vi "Day 23.vi"() -> ()   [LabVIEW 2021]
uses:
  Hallway Positions Enum.ctl
  Room Enum.ctl
  Zone Enum.ctl
  Position Cluster.ctl
  Amphipod Enum.ctl
  <vilib>/Utility/miscctls.llb/LVMapReplaceAction.ctl
  <vilib>/Utility/file.llb/Read Delimited Spreadsheet (string).vi
panel:
  out "Energy out":i32
  out "State out":map{T1, T2[]}(c390)
  out "Map":map{T1, T2[]}(c390)
  out "subarray":string[](array[string])
  in  "Input File":enum32{"example input", "input"}(radio)
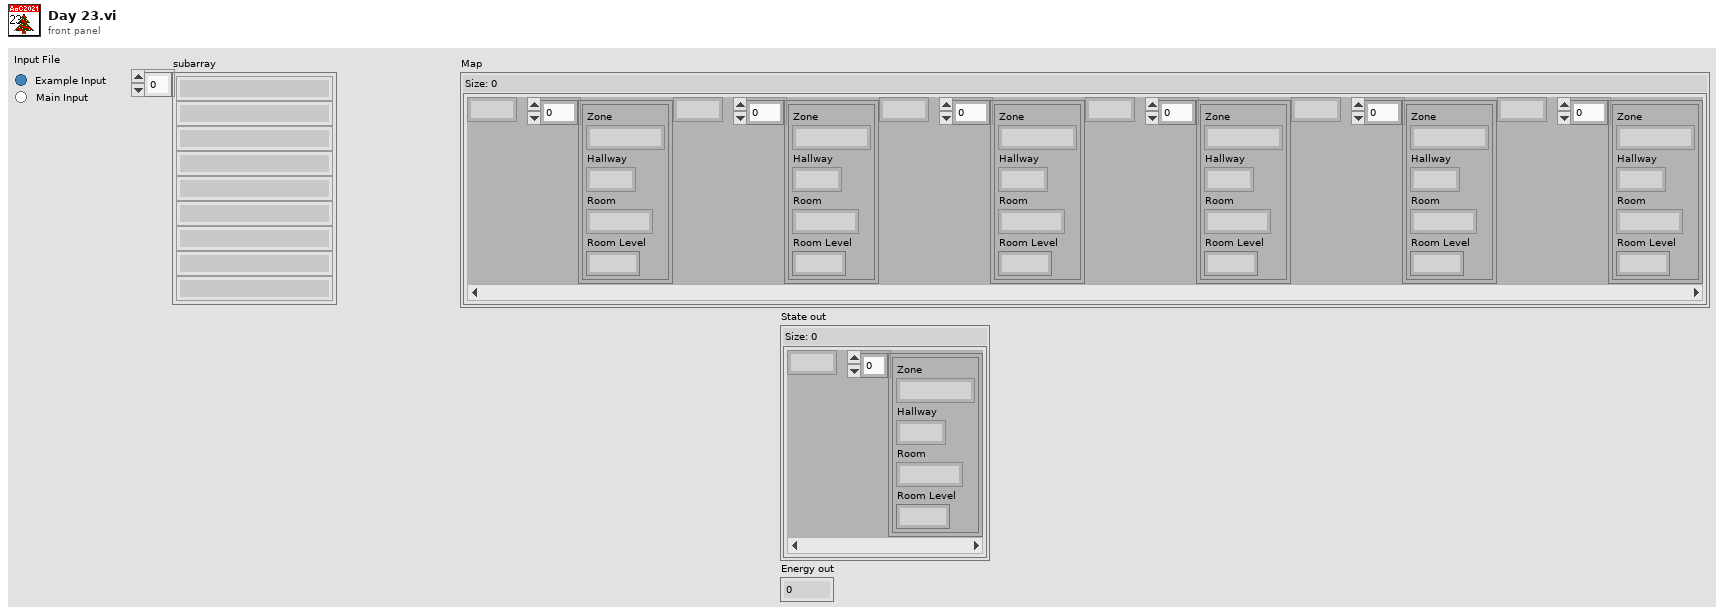
[diagram p1: front panel]
types:
  T1 = typedef "Amphipod Enum.ctl" = enum16{"A", "B", "C", "D"}
  T2 = typedef "Position Cluster.ctl" = cluster{"Zone":T3, "Hallway":T4, "Room":T5, "Room Level":i32}
  T3 = typedef "Zone Enum.ctl" = enum16{"Hallway", "Room"}
  T4 = typedef "Hallway Positions Enum.ctl" = enum16{"H1", "H2", "D3", "H4", "D5", "H6", "D7", "H8", "D9", "H10", "H11"}
  T5 = typedef "Room Enum.ctl" = enum16{"Room A", "Room B", "Room C", "Room D"}
  T6 = typedef "LVMapReplaceAction.ctl" = enum32{"Modify Entry only if found", "Add or Modify Entry", "Delete Entry"}
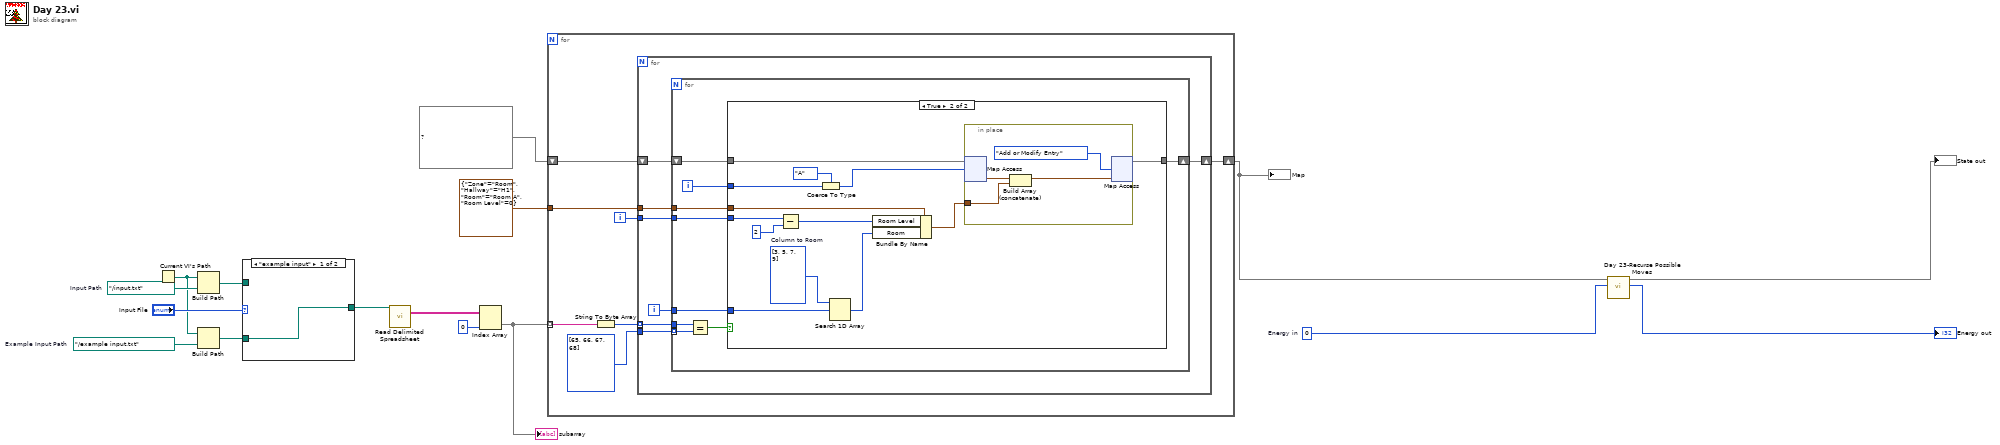
[diagram p0: block diagram]
diagram:
  w2 = 0  # Energy in
  w15 = path "../example input.txt"  # Example Input Path
  w16 = path "../input.txt"  # Input Path
  n1 = Current VI's Path() -> (path=w10:path)
  n2 = Build Path(base path=w10, name or relative path=w16) -> (appended path=w13:path)
  n3 = Build Path(base path=w10, name or relative path=w15) -> (appended path=w12:path)
  n4 = case shown="\"example input\"" "Input File" {
    tunnel: w13 -> [_ w18]
    tunnel: w12 -> [w17 _]
    tunnel: [w17 w18] -> w11
    frame "example input" {
    }
    frame "input" {
    }
  }
  n5 = call-poly <vilib>:"Read Delimited Spreadsheet.vi"("file path (dialog if empty)"=w11) -> ("all rows"=w9:string[][])  [unwired: 9 in, 5 out]
  n6 = Index Array(array=w9, index (col)=0 ("disabled index (col)")) -> (element=w7:string[])  [unwired: 1 in]
  "subarray" <- w7
  n7 = for {
    tunnel: w7 -> [w25] mode=indexing
    tunnel: T2 {"Zone"=enum."Room", "Hallway"=enum."H1", "Room"=enum."Room A", "Room Level"=0} -> [w22]
    shift-right: [w21] -> w5
    shift-left: map{T1, T2[]} {} ("map in") -> [w20]
    i -> [w19]
    n8 = String To Byte Array(string=w25) -> (unsigned byte array=w24:u8[])
    n9 = for {
      tunnel: w24 -> [w32] mode=indexing
      tunnel: i32[] [65, 66, 67, 68] -> [w31]
      tunnel: w22 -> [w30]
      shift-right: [w29] -> w21
      shift-left: w20 -> [w28]
      tunnel: w19 -> [w27]
      i -> [w26]
      n10 = for {
        tunnel: w32 -> [w41]
        tunnel: w31 -> [w40] mode=indexing
        tunnel: w30 -> [w37]
        shift-right: [w39] -> w29
        shift-left: w28 -> [w38]
        tunnel: w27 -> [w34]
        tunnel: w26 -> [w33]
        i -> [w35]
        n11 = Equal?(x=w41, y=w40) -> (x = y?=w36:bool)
        n12 = case shown="True" w36 {
          tunnel: [w42 w46] -> w39
          tunnel: w38 -> [w42 w44]
          tunnel: w37 -> [_ w55]
          tunnel: w35 -> [_ w48]
          tunnel: w34 -> [_ w54]
          tunnel: w33 -> [_ w50]
          frame False {
          }
          frame True {
            w51 = i32[] [3, 5, 7, 9]  # Column to Room
            n13 = Subtract(x=w54, y=2) -> (x-y=w52:i32)
            n14 = Coerce To Type(0:w48, 1:Amphipod_Enum."A" ("Amphipod Enum")) -> (2:w43:T1)
            n15 = Search 1D Array(1D array=w51, element=w50) -> (index of element=w49:i32)  [unwired: 1 in]
            n16 = Bundle By Name(cluster=w55, "Room Level"=w52, "Room"=w49) -> (w45:T2)
            n17 = in-place {
              in-place-border: w45 -> [w59]
              n18 = in-place-map #1(w44, w43) -> (w58:T2[])  [unwired: 1 in, 1 out]
              n19 = Build Array (concatenate)(w58, w59) -> (w57:T2[])
              n20 = in-place-map #1(w57, LVMapReplaceAction."Add or Modify Entry" ("action")) -> (w46:map{T1, T2[]})  [unwired: 2 out]
            }
          }
        }
      }
    }
  }
  "Map" <- w5
  n21 = call "Day 23-Recurse Possible Moves.vi"("Energy in"=w2, "State in"=w5) -> ("Energy out"=→"Energy out":i32, "State out"=→"State out":map{T1, T2[]})  [unwired: 8 in]
